vi "RGBtoGRB.vi"(1 "Color (RGB)":u32(colorbox)) -> (0 "Color (GRB)":u32(colorbox))   [LabVIEW 2019]
doc: "Converts RGB colors into GRB colors for the LED strips."
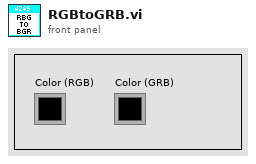
[diagram p1: front panel]
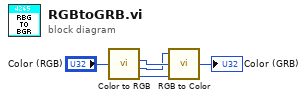
[diagram p0: block diagram]
diagram:
  n1 = call <vilib>:"Color to RGB.vi"("Color"="Color (RGB)") -> ("R"=w3:u8, "G"=w2:u8, "B"=w1:u8)  [unwired: 1 out]
  n2 = call <vilib>:"RGB to Color.vi"("B"=w1, "G"=w3, "R"=w2) -> ("Color"=→"Color (GRB)":u32)
